vi "EyeHistogram.vi"() -> ()   [LabVIEW 2022 SP3]
uses:
  <vilib>/Analysis/NI_AALPro.lvlib
panel:
  out "3 freq bins for histogram":T1(graph)=[{"X Values"=[1.027898243958004, 3.052279300012354, 5.0766603560667045, 7.101041412121054, 9.125422468175405, 11.149803524229755, 13.174184580284104, 15.198565636338454, 17.222946692392803, 19.247327748447155, 21.271708804501504, 23.296089860555856, 25.320470916610205, 27.344851972664554, 29.369233028718906, 31.393614084773255, 33.41799514082761, 35.44237619688195, 37.466757252936304, 39.49113830899066, 41.515519365045, 43.539900421099354, 45.564281477153706, 47.58866253320806, 49.6130435892624, 51.637424645316756, 53.66180570137111, 55.68618675742545, 57.710567813479805, 59.73494886953416, 61.7593299255885, 63.783710981642855, 65.80809203769721, 67.83247309375156, 69.85685414980591, 71.88123520586025, 73.9056162619146, 75.92999731796895, 77.9543783740233, 79.97875943007766], "Histogram: h(x)"=[109, 332, 533, 743, 862, 986, 991, 941, 914, 870, 785, 711, 657, 608, 496, 449, 392, 338, 324, 213, 181, 138, 97, 96, 77, 45, 37, 38, 31, 22, 20, 13, 10, 11, 17, 8, 7, 5, 1, 2]}, {"X Values"=[3.3829204156339503, 5.6173167979244845, 7.85171318021502, 10.086109562505554, 12.32050594479609, 14.554902327086623, 16.789298709377157, 19.023695091667694, 21.258091473958228, 23.49248785624876, 25.726884238539295, 27.961280620829832, 30.195677003120366, 32.4300733854109, 34.66446976770143, 36.89886614999197, 39.1332625322825, 41.36765891457304, 43.602055296863576, 45.83645167915411, 48.07084806144464, 50.30524444373518, 52.53964082602571, 54.774037208316244, 57.00843359060678, 59.24282997289732, 61.47722635518785, 63.711622737478386, 65.94601911976892, 68.18041550205946, 70.41481188434999, 72.64920826664053, 74.88360464893105, 77.1180010312216, 79.35239741351212, 81.58679379580266, 83.82119017809319, 86.05558656038373, 88.28998294267427, 90.5243793249648], "Histogram: h(x)"=[8, 19, 104, 210, 372, 696, 919, 858, 1015, 1029, 1012, 1012, 941, 769, 774, 756, 611, 547, 327, 231, 185, 151, 123, 84, 56, 37, 24, 26, 25, 34, 43, 28, 16, 15, 13, 11, 8, 8, 8, 5]}]
  out "5 freq bins in histogram":T1(graph)=[{"X Values"=[1.027898243958004, 3.052279300012354, 5.0766603560667045, 7.101041412121054, 9.125422468175405, 11.149803524229755, 13.174184580284104, 15.198565636338454, 17.222946692392803, 19.247327748447155, 21.271708804501504, 23.296089860555856, 25.320470916610205, 27.344851972664554, 29.369233028718906, 31.393614084773255, 33.41799514082761, 35.44237619688195, 37.466757252936304, 39.49113830899066, 41.515519365045, 43.539900421099354, 45.564281477153706, 47.58866253320806, 49.6130435892624, 51.637424645316756, 53.66180570137111, 55.68618675742545, 57.710567813479805, 59.73494886953416, 61.7593299255885, 63.783710981642855, 65.80809203769721, 67.83247309375156, 69.85685414980591, 71.88123520586025, 73.9056162619146, 75.92999731796895, 77.9543783740233, 79.97875943007766], "Histogram: h(x)"=[109, 332, 533, 743, 862, 986, 991, 941, 914, 870, 785, 711, 657, 608, 496, 449, 392, 338, 324, 213, 181, 138, 97, 96, 77, 45, 37, 38, 31, 22, 20, 13, 10, 11, 17, 8, 7, 5, 1, 2]}, {"X Values"=[12.28382444526186, 14.539669020364993, 16.795513595468123, 19.051358170571255, 21.307202745674385, 23.563047320777518, 25.818891895880647, 28.07473647098378, 30.33058104608691, 32.58642562119004, 34.84227019629317, 37.098114771396304, 39.35395934649944, 41.60980392160256, 43.865648496705695, 46.12149307180883, 48.37733764691196, 50.63318222201509, 52.88902679711822, 55.14487137222135, 57.400715947324485, 59.65656052242761, 61.912405097530744, 64.16824967263388, 66.424094247737, 68.67993882284014, 70.93578339794327, 73.1916279730464, 75.44747254814953, 77.70331712325266, 79.9591616983558, 82.21500627345893, 84.47085084856205, 86.72669542366519, 88.98253999876832, 91.23838457387144, 93.49422914897458, 95.75007372407771, 98.00591829918085, 100.26176287428397], "Histogram: h(x)"=[53, 116, 161, 471, 620, 575, 897, 985, 973, 910, 954, 796, 854, 793, 733, 582, 455, 460, 316, 315, 205, 196, 144, 79, 54, 62, 45, 46, 58, 35, 29, 25, 33, 19, 17, 9, 14, 7, 7, 7]}]
  out "sum of bins after sector conversion":dbl[][](graph)
  out "sum of bins before sector conversion":dbl[][](graph)
  out "before":dbl[][](graph)
  out "bin 3":dbl[][](graph)
  out "bin 2":dbl[][](graph)
  out "bin 1":dbl[][](graph)
  in  "bin envelopes":dbl[][][](array[numeric]) format="%.2f"
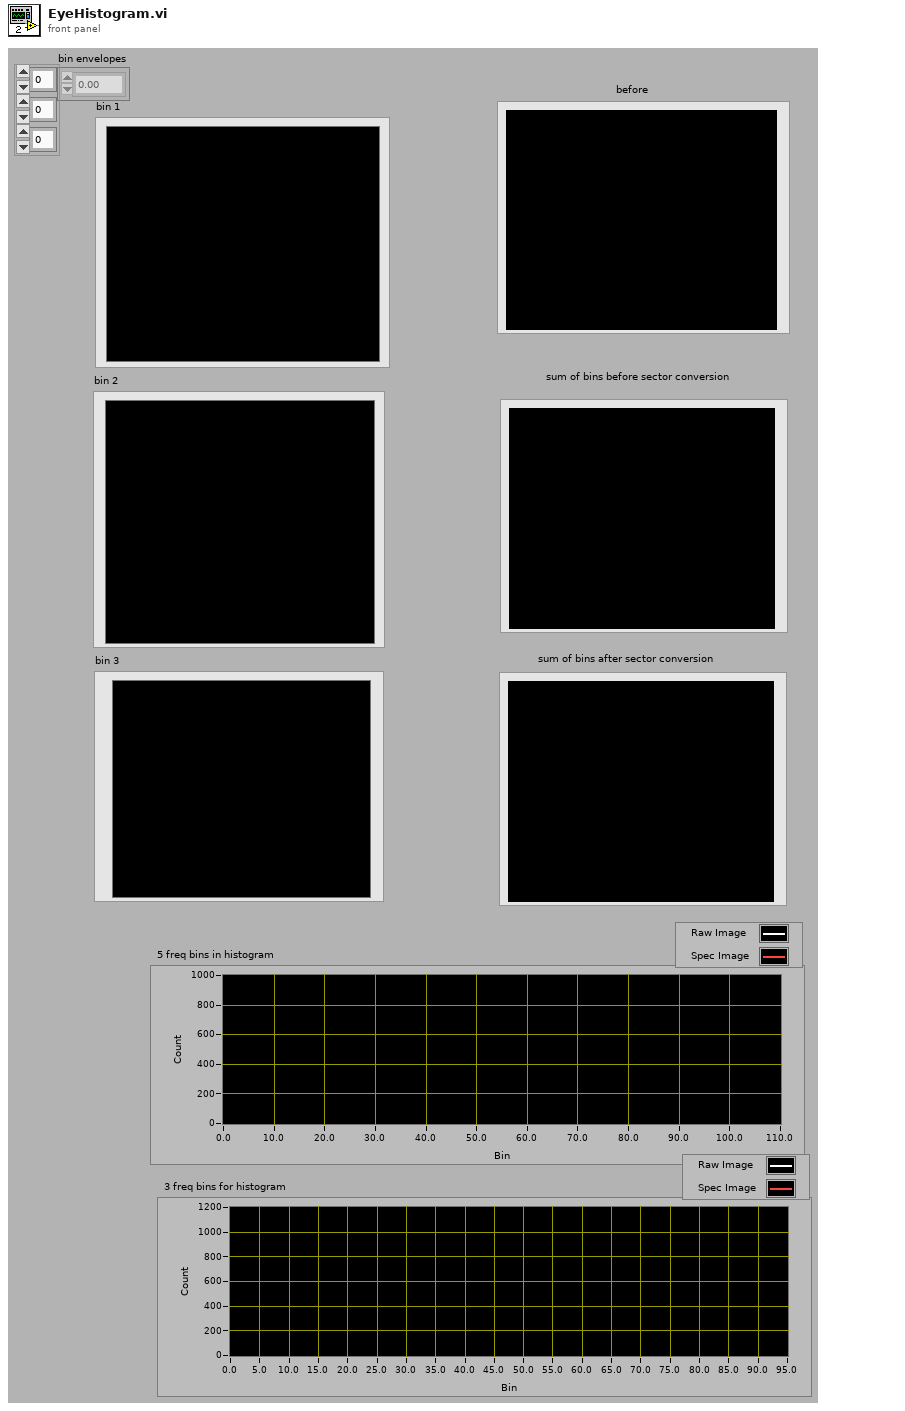
[diagram p1: front panel]
types:
  T1 = cluster{"X Values":dbl[], "Histogram: h(x)":i32[]}[]
  T2 = cluster{"delay":sgl, "pivot distance":sgl, "sector scan angle":sgl, "operator":string, "Scan Mode":string, "location":string}
  T3 = cluster{"# rf points per line":u16, "# lines per scan":u16, "sample rate MHz":u16, "# A/D bits":i16, "# bytes per A/D":u16, "TGC Flag":u16, "A/D Type":string}
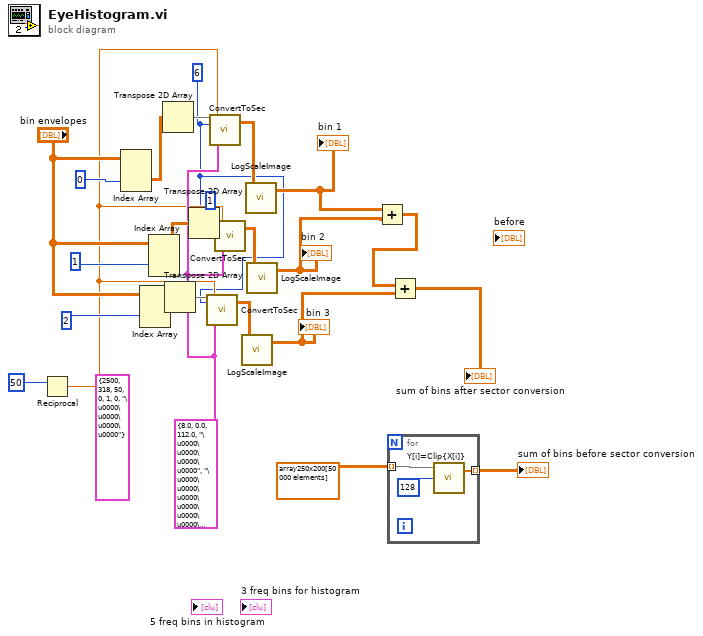
[diagram p0: block diagram]
diagram:
  w15 = T2 {"delay"=8.0, "pivot distance"=0.0, "sector scan angle"=112.0, "operator"="\u0000\u0000\u0000\u0000", "Scan Mode"="\u0000\u0000\u0000\u0000\u0000\u0000\u0000", "location"="\u0000\u0000\u0000\u0000\u0000\u0000\u0000\u0000\u0000"} ("Scan Info")
  (unwired) T3 {"# rf points per line"=2500, "# lines per scan"=318, "sample rate MHz"=50, "# A/D bits"=0, "# bytes per A/D"=1, "TGC Flag"=0, "A/D Type"="\u0000\u0000\u0000\u0000"} ("A/D info")
  w1 = 6
  (unwired) 1
  n1 = Reciprocal(x=50) -> (1/x=w12:dbl)
  n2 = Index Array(array="bin envelopes", index (dim 1)=0) -> (element=w13:dbl[][])  [unwired: 2 in]
  n3 = Index Array(array="bin envelopes", index (dim 1)=2) -> (element=w18:dbl[][])  [unwired: 2 in]
  n4 = Index Array(array="bin envelopes", index (dim 1)=1) -> (element=w19:dbl[][])  [unwired: 2 in]
  n5 = Transpose 2D Array(2D array=w13) -> (transposed array=w11:dbl[][])
  n6 = Transpose 2D Array(2D array=w18) -> (transposed array=w9:dbl[][])
  n7 = Transpose 2D Array(2D array=w19) -> (transposed array=w10:dbl[][])
  n8 = call "ConvertToSec.vi"("raw image data in"=w9, "reduce pts by factor of"=w1, "Time between rf pts\nmicros"=w12, "Scan Info"=w15) -> ("raw sector out"=w17:dbl[][])  [unwired: 7 in, 8 out]
  n9 = call "ConvertToSec.vi"("raw image data in"=w11, "reduce pts by factor of"=w1, "Time between rf pts\nmicros"=w12, "Scan Info"=w15) -> ("raw sector out"=w20:dbl[][])  [unwired: 7 in, 8 out]
  n10 = call "ConvertToSec.vi"("raw image data in"=w10, "reduce pts by factor of"=w1, "Time between rf pts\nmicros"=w12, "Scan Info"=w15) -> ("raw sector out"=w16:dbl[][])  [unwired: 7 in, 8 out]
  n11 = call "LogScaleImage.vi"("input array"=w17) -> ("log scale image"=w6:dbl[][])  [unwired: 1 in, 1 out]
  "bin 3" <- w6
  n12 = call "LogScaleImage.vi"("input array"=w20) -> ("log scale image"=w8:dbl[][])  [unwired: 1 in, 1 out]
  "bin 1" <- w8
  n13 = call "LogScaleImage.vi"("input array"=w16) -> ("log scale image"=w7:dbl[][])  [unwired: 1 in, 1 out]
  "bin 2" <- w7
  n14 = Add(x=w8, y=w7) -> (x+y=w5:dbl[][])
  n15 = for {
    tunnel: dbl[][] array250x200[50000 elements] ("sum of bins before sector conversion") -> [w27] mode=indexing
    tunnel: [w25] -> w2 mode=indexing
    n16 = call <vilib>:"Y[i]=Clip{X[i]}.vi"("upper limit"=128, "Input Array"=w27) -> ("Clipped Array"=w25:dbl[])  [unwired: 1 in, 1 out]
  }
  "sum of bins before sector conversion" <- w2
  n17 = Add(x=w5, y=w6) -> (x+y=→"sum of bins after sector conversion":dbl[][])
